vi "MultiDiagramStructureToJson.vi"(0 "MultiDiagramStructure in":refnum<vi>, 1 "Relative Bounds":cluster{"x":i32, "y":i32, "w":i32, "h":i32}, 2 "Current Path":path, 3 "Origin Path":path, 4 "Component Idx":i32, 5 "error in (no error)":errorcluster) -> (15 "JSON":string, 19 "error IO":errorcluster)   [LabVIEW 2017]
doc: "Creates a JSON for a Multidiagram Structure"
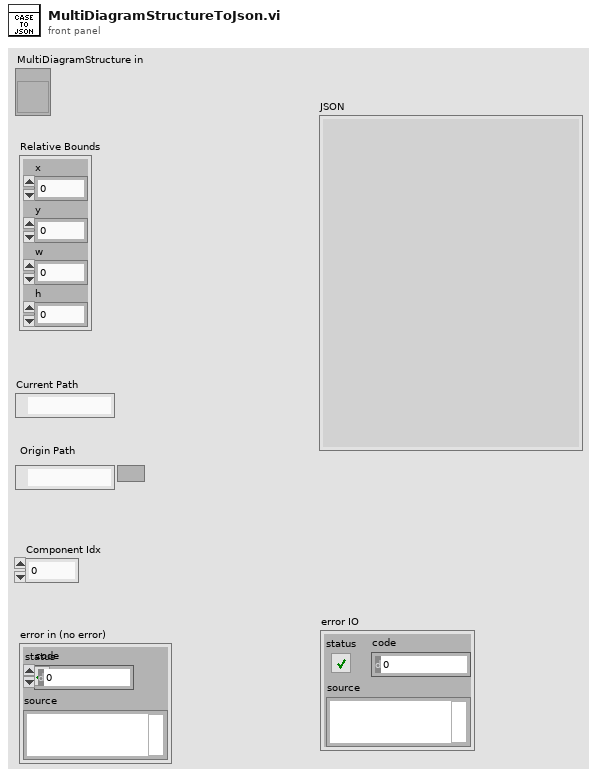
[diagram p1: front panel]
types:
  T1 = typedef "LVRectTypeDef.ctl" = cluster{"Left":i16, "Top":i16, "Right":i16, "Bottom":i16}
  T2 = typedef "imagedata.ctl" = cluster{"image type":i32, "image depth":i32, "image":u8[], "mask":u8[], "colors":u32[], "Rectangle":cluster{"left":i16, "top":i16, "right":i16, "bottom":i16}}
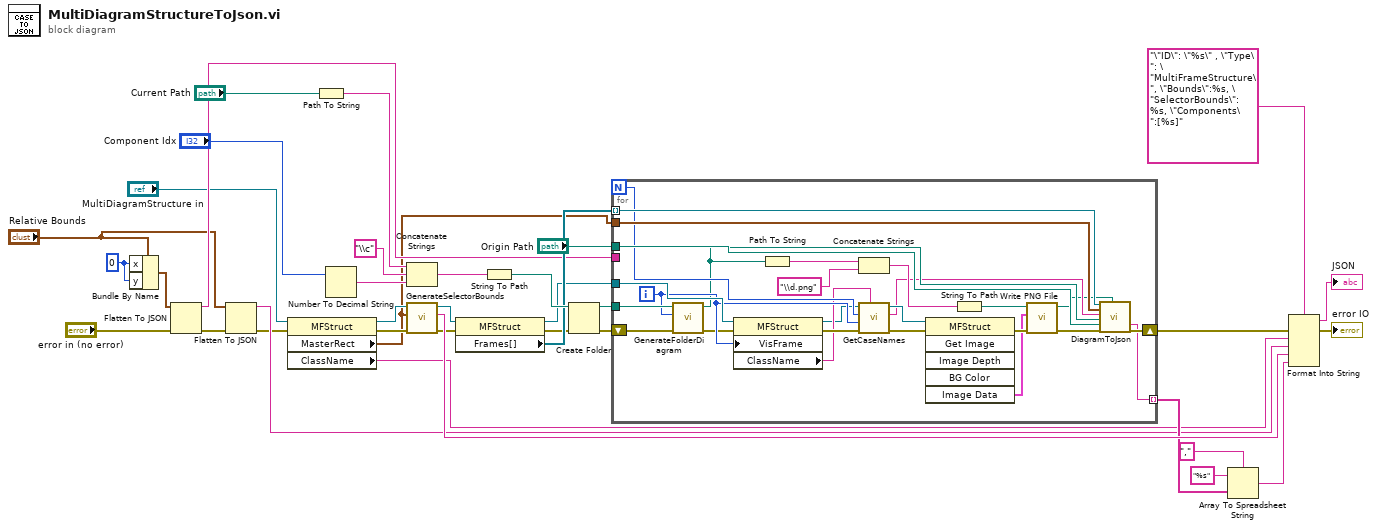
[diagram p0: block diagram]
diagram:
  w10 = 0 ("x")
  n1 = Bundle By Name(cluster="Relative Bounds", "x"=w10, "y"=w10) -> (w23:cluster{"x":i32, "y":i32, "w":i32, "h":i32})
  n2 = Flatten To JSON(anything=w23, error in (no error)="error in (no error)") -> (JSON string=w22:string, 11:w7:errorcluster)  [unwired: 1 in]
  n3 = Flatten To JSON(anything="Relative Bounds", error in (no error)=w7) -> (JSON string=w16:string, 11:w6:errorcluster)  [unwired: 1 in]
  n4 = property class="MFStruct"(reference="MultiDiagramStructure in", error in=w6) -> (reference out=w13:refnum<vi>, error out=w9:errorcluster, "MasterRect"=w2:T1, "ClassName"=w1:string)
  n5 = Path To String(path="Current Path") -> (string=w17:string)
  n6 = Number To Decimal String(number="Component Idx") -> (decimal integer string=w32:string)  [unwired: 1 in]
  n7 = Concatenate Strings(w17, "\\c" ("string"), w32) -> (w30:string)
  n8 = call "GenerateSelectorBounds.vi"("error in (no error)"=w9, "Master Bounds Rect"=w2, "MultiFrameStructure in"=w13) -> ("error out"=w12:errorcluster, "JSON string"=w27:string, "reference out"=w33:refnum<vi>)  [unwired: 6 in]
  n9 = property class="MFStruct"(reference=w33, error in=w12) -> (reference out=w25:refnum<vi>, error out=w4:errorcluster, "Frames[]"=w26:refnum<vi>[])
  n10 = String To Path(string=w30) -> (path=w29:path)
  n11 = Create Folder(path (use dialog)=w29, error in=w4) -> (created path=w24:path, error out=w3:errorcluster)  [unwired: 1 in, 1 out]
  n12 = for {
    N -> [w52]
    tunnel: w26 -> [w58] mode=indexing
    tunnel: w25 -> [w63]
    tunnel: w24 -> [w62]
    tunnel: w2 -> [w55]
    tunnel: "Origin Path" -> [w54]
    tunnel: w22 -> [_]
    tunnel: [w38] -> w19 mode=indexing
    shift-right: [w39] -> w15
    shift-left: w3 -> [w43]
    i -> [w56]
    n13 = call "GenerateFolderDiagram.vi"("error in"=w43, "Numeric"=w56, "created path in"=w62) -> ("error out"=w42:errorcluster, "created path out"=w44:path)  [unwired: 7 in]
    n14 = property class="MFStruct"(reference=w63, error in=w42, "VisFrame"=w56) -> (reference out=w49:refnum<vi>, error out=w57:errorcluster, "ClassName"=w50:string)
    n15 = Path To String(path=w44) -> (string=w53:string)
    n16 = Concatenate Strings(w53, "\\d.png" ("string")) -> (w60:string)
    n17 = call "GetCaseNames.vi"("ClassName"=w50, "error in (no error)"=w57, "Numeric 2"=w56, "Numeric"=w52, "MultiFrameStructure in"=w49) -> ("error out"=w47:errorcluster, "String"=w41:string, "MultiFrameStructure out"=w48:refnum<vi>)  [unwired: 4 in]
    n18 = invoke class="MFStruct" method="Get Image"(reference=w48, error in=w47) -> (error out=w46:errorcluster, "Image Data"=w45:T2)  [unwired: 4 in, 4 out]
    n19 = String To Path(string=w60) -> (path=w59:path)
    n20 = call <vilib>:"Write PNG File.vi"("error in (no error)"=w46, "image data"=w45, "path to PNG file"=w59) -> ("error out"=w51:errorcluster, "path"=w40:path)  [unwired: 7 in]
    n21 = call "DiagramToJson.vi"("GObj in"=w58, "Owner Bounds"=w55, "ID"=w41, "Current Path"=w44, "Origin Path"=w54, "error in (no error)"=w51, "Image Path"=w40) -> ("JSON (out)"=w38:string, "error out"=w39:errorcluster)  [unwired: 10 in, 1 out]
  }
  n22 = Array To Spreadsheet String(delimiter (Tab)=",", array=w19, 3:"%s" ("format string")) -> (spreadsheet string=w18:string)
  n23 = Format Into String(format string="\"ID\": \"%s\" , \"Type\": \"MultiFrameStructure\", \"Bounds\":%s, \"SelectorBounds\": %s, \"Components\":[%s]", error in=w15, w1, w16, w27, w18) -> (resulting string=→"JSON":string, error out=→"error IO":errorcluster)  [unwired: 1 in]
